vi "tt20_get_histogram.vi"(8 "error in (no error)":errorcluster, 11 "tt20 in":refnum<class "tt20.lvclass">) -> (0 "error out":errorcluster, 2 "histogram":cluster{dbl[], dbl[]}[](array[cluster]), 3 "tt20 out":refnum<class "tt20.lvclass">)   [LabVIEW 2015, in "tt20.lvclass"]
uses:
  tt20.lvclass
  tt20.lvclass/tt20.ctl
  C:/Users/MX-Microscope/Documents/LabVIEW Data/lvoop_campus_2018/Detector_Class/Swabian/time_tagger_vis/TTCSharp32.dll
  time_tagger_vis/TTCSharp32.dll
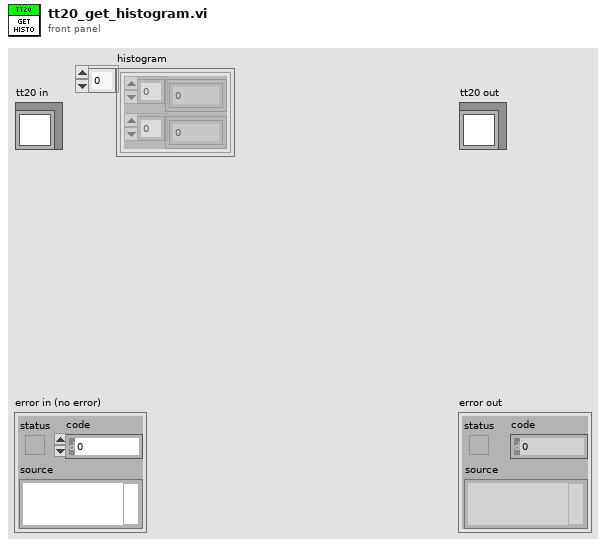
[diagram p1: front panel]
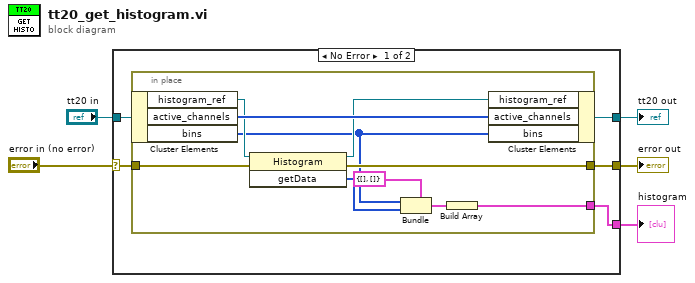
[diagram p0: block diagram]
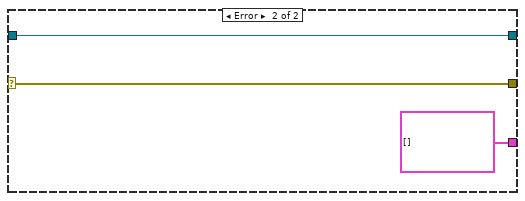
[diagram p2: hidden frame]
diagram:
  n1 = case shown="No Error" "error in (no error)" {
    selector: "error in (no error)" -> [w9 w23]
    tunnel: "tt20 in" -> [w10 w22]
    tunnel: [w8 w22] -> w3
    tunnel: [w7 w23] -> w2
    tunnel: [w6 cluster{dbl[], dbl[]}[] []] -> w1
    frame No Error {
      n2 = in-place {
        in-place-border: w9 -> [w17]
        in-place-border: [w16] -> w7
        in-place-border: [w12] -> w6
        n3 = in-place-cluster #1(w10) -> ("histogram_ref"=w19:refnum<k24>, "active_channels"=w20:u32[], "bins"=w11:i64[])
        n4 = invoke class="Histogram" method="getData"(reference=w19, error in=w17) -> (reference out=w18:refnum<k24>, error out=w16:errorcluster, "getData"=w15:i32[])  [unwired: 1 in]
        n5 = Bundle(cluster=cluster{dbl[], dbl[]} {[], []} ("element"), w11, w15) -> (w13:cluster{dbl[], dbl[]})
        n6 = Build Array(w13) -> (w12:cluster{dbl[], dbl[]}[])
        n7 = in-place-cluster #1("histogram_ref"=w18, "active_channels"=w20, "bins"=w11) -> (w8:refnum<class "tt20.lvclass">)
      }
    }
    frame Error {
    }
  }
  "error out" <- w2
  "tt20 out" <- w3
  "histogram" <- w1
